vi "norm (SubVI).vi"(9 "OK Button":bool, 10 "std":dbl, 11 "mean":dbl) -> (2 "stOut":dbl, 3 "meanOut":dbl)   [LabVIEW 2011]
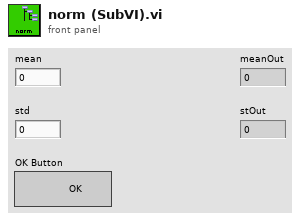
[diagram p1: front panel]
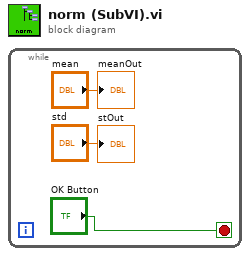
[diagram p0: block diagram]
diagram:
  n1 = while {
    stop <- "OK Button" stop-if-true
    "meanOut" <- "mean"
    "stOut" <- "std"
  }
